vi "Read Config.vi"(8 "error in (no error)":errorcluster, 9 "Re-Init?":bool, 10 "ICM File In":path, 11 "No-Op in":refnum<class "No-Op Output.lvclass">) -> (0 "error out":errorcluster, 3 "No-Op out":refnum<class "No-Op Output.lvclass">)   [LabVIEW 2018, in "No-Op Output.lvclass"]
doc: "Single Channel.lvclass:Read Config.vi\n\nThis VI reads the Single Channel Class parameters from the ICM configuration file.\n\nInstrument Communication Module Version 1.0\nOctober, 2020 Original Code Consulting Davita Bird\n www.originalcode.com"
uses:
  No-Op Output.lvclass
  No-Op Output.lvclass/No-Op Output.ctl
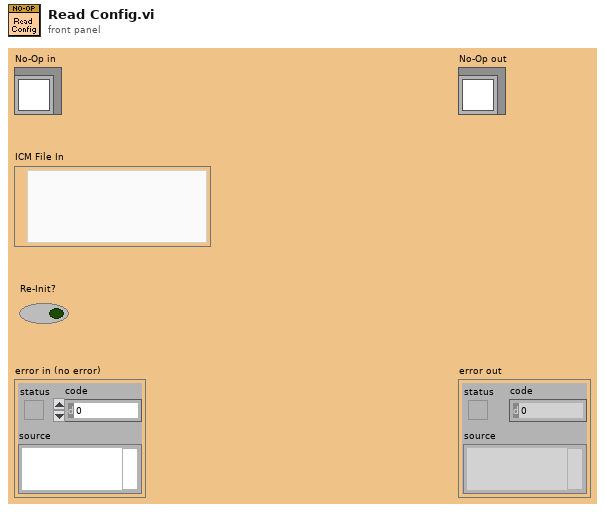
[diagram p1: front panel]
types:
  T1 = typedef "No-Op.ctl" = cluster{"Channels":string[], "Enabled":bool[], "Initial Values":dbl[], "Set Initial Values At Startup?":bool}
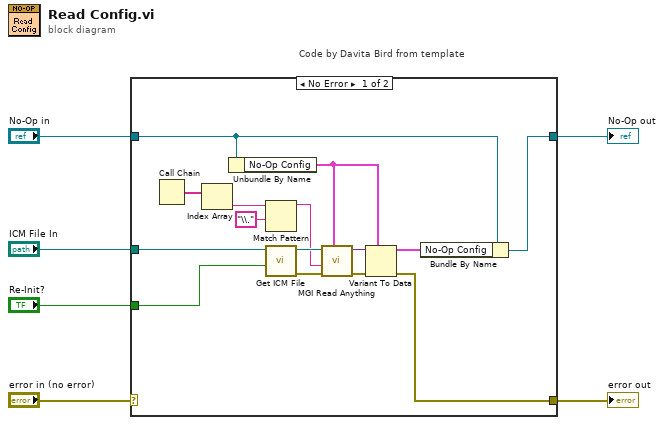
[diagram p0: block diagram]
diagram:
  n1 = case "Code by Davita Bird from template" shown="No Error" "error in (no error)" {
    selector: "error in (no error)" -> [_ w23]
    tunnel: [w13 w23] -> w5
    tunnel: [w9 w22] -> w3
    tunnel: "No-Op in" -> [w11 w22]
    tunnel: "ICM File In" -> [w8 _]
    tunnel: "Re-Init?" -> [w7 _]
    frame No Error {
      n2 = Call Chain() -> (call chain=w18:string[])
      n3 = Index Array(array=w18) -> (element=w19:string)  [unwired: 1 in]
      n4 = Unbundle By Name(w11) -> ("No-Op Config"=w10:T1)
      n5 = Match Pattern(string=w19, regular expression="\\.") -> (before substring=w16:string)  [unwired: 1 in, 3 out]
      n6 = call "Get ICM File.vi"("Re-Init?"=w7, "ICM File In"=w8) -> ("error out"=w20:errorcluster, "ICM File"=w21:path)  [unwired: 8 in]
      n7 = call <userlib>:"MGI Read Anything.vi"("Type of Anything"=w10, "Error In"=w20, "Section Name (Name of \"Type of Anything\")"=w16, "Path (dialog)"=w21) -> ("Error Out"=w14:errorcluster, "Anything"=w15:variant)  [unwired: 4 in, 2 out]
      n8 = Variant To Data(error in=w14, type=w10, Variant=w15) -> (data=w12:T1, error out=w13:errorcluster)
      n9 = Bundle By Name(cluster=w11, "No-Op Config"=w12) -> (w9:refnum<class "No-Op Output.lvclass">)
    }
    frame Error {
    }
  }
  "error out" <- w5
  "No-Op out" <- w3
